vi "Scan Hydra - Check.vi"(2 "error in":errorcluster) -> (0 "error out":errorcluster, 1 "next scan":dbl[](array[numeric]) format="%.2f")   [LabVIEW 2019]
uses:
  Global Variables/Global_Variables.vi
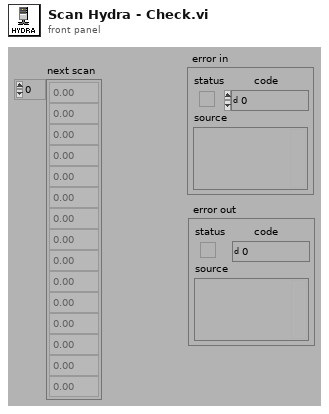
[diagram p1: front panel]
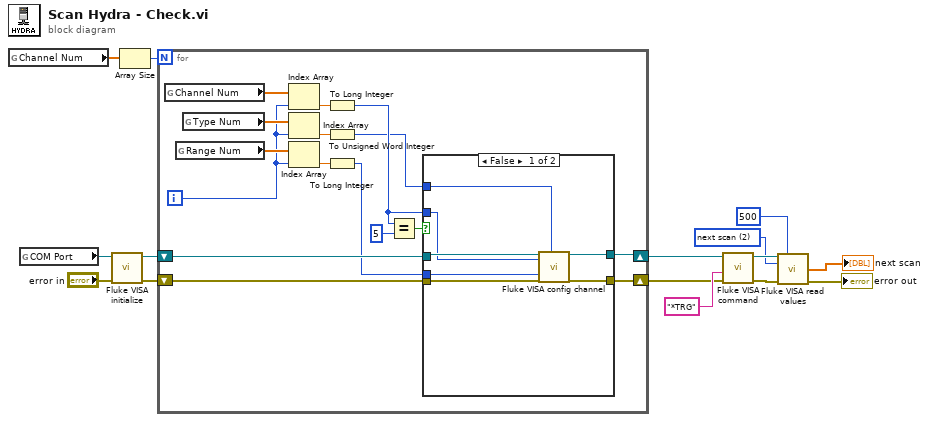
[diagram p0: block diagram]
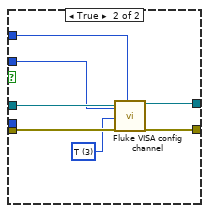
[diagram p2: hidden frame]
diagram:
  w10 = 2 items=["min, max, & last", "monitor value", "next scan", "current total"] ("values to read")
  n1 = global read "Global_Variables.vi" "Channel Num"() -> (w6:dbl[])
  n2 = global read "Global_Variables.vi" "COM Port"() -> (w7:refnum<visa-resource-name>)
  n3 = call "Fluke VISA initialize.vi"("error in (no error)"="error in", "Hydra VISA in"=w7) -> ("error out"=w3:errorcluster, "Hydra VISA out"=w4:refnum<visa-resource-name>)  [unwired: 3 in, 1 out]
  n4 = Array Size(array=w6) -> (size(s)=w5:i32)
  n5 = for {
    N: w5 -> [_]
    shift-right: [w20] -> w1
    shift-left: w4 -> [w23]
    shift-right: [w19] -> w2
    shift-left: w3 -> [w22]
    i -> [w28]
    n6 = global read "Global_Variables.vi" "Channel Num"() -> (w31:dbl[])
    n7 = global read "Global_Variables.vi" "Range Num"() -> (w29:dbl[])
    n8 = global read "Global_Variables.vi" "Type Num"() -> (w30:dbl[])
    n9 = Index Array(array=w31, index=w28) -> (element=w27:dbl)
    n10 = Index Array(array=w30, index=w28) -> (element=w26:dbl)
    n11 = Index Array(array=w29, index=w28) -> (element=w25:dbl)
    n12 = To Long Integer(number=w27) -> (32bit integer=w21:i32)
    n13 = To Unsigned Word Integer(number=w26) -> (unsigned 16bit integer=w18:u16)
    n14 = To Long Integer(number=w25) -> (32bit integer=w17:i32)
    n15 = Equal?(x=w21, y=5) -> (x = y?=w24:bool)
    n16 = case shown="False" w24 {
      tunnel: w23 -> [w37 w44]
      tunnel: w22 -> [w38 w45]
      tunnel: w21 -> [w34 w43]
      tunnel: [w32 w42] -> w20
      tunnel: [w33 w41] -> w19
      tunnel: w18 -> [w35 w40]
      tunnel: w17 -> [w36 _]
      frame False {
        n17 = call "Fluke VISA config channel.vi"("Hydra VISA in"=w37, "channel"=w34, "range (auto:0)"=w36, "error in (no error)"=w38, "function (off:0)"=w35) -> ("Hydra VISA out"=w32:refnum<visa-resource-name>, "error out"=w33:errorcluster)  [unwired: 13 in]
      }
      frame True {
        w39 = 3 items=["J", "K", "E", "T", "N", "R", "S", "B", "C"] ("thermocouple (J:0)")
        n18 = call "Fluke VISA config channel.vi"("Hydra VISA in"=w44, "channel"=w43, "thermocouple (J:0)"=w39, "error in (no error)"=w45, "function (off:0)"=w40) -> ("Hydra VISA out"=w42:refnum<visa-resource-name>, "error out"=w41:errorcluster)  [unwired: 13 in]
      }
    }
  }
  n19 = call "Fluke VISA command.vi"("error in (no error)"=w2, "Single Command"="*TRG", "Hydra VISA in"=w1) -> ("error out"=w13:errorcluster, "Hydra VISA out"=w14:refnum<visa-resource-name>)  [unwired: 3 in, 2 out]
  n20 = call "Fluke VISA read values.vi"("Hydra VISA in"=w14, "Byte Count"=u32 500, "values to read"=w10, "error in (no error)"=w13) -> ("next scan"=→"next scan":dbl[], "error out"=→"error out":errorcluster)  [unwired: 4 in, 6 out]
